vi "Util.Cmprs.LZW.CU_CompressUncompress__ogtk.vi"(8 "error in (no error)":errorcluster, 9 "LZWBits":i32, 10 "Data":u8[](array[numeric]) format="%.0x", 11 "Compress/Decompress (T/F)":bool) -> (0 "error out":errorcluster, 2 "Data out":u8[](array[numeric]) format="%.0x")   [LabVIEW 2020]
panel:
  # "LZW.CU_CompressUncompress.vi\n\nCompresses or Uncompresses data-stream according to the \"Lempel-Ziv-Welch\" compression algorithm\n\nPlease visit http://www.OpenG.org to learn about the\nOpen Source LabVIEW software movement.\n\nNOTICE -- YOU MUST LEAVE THIS NOTICE IN PLACE.  PER THE TERMS OF THE LICENSE BELOW, YOU MAY SUBLICENSE THIS SOFTWARE \nIN ANY WAY THAT DOES NOT CONFLICT WITH THIS LICENSE.\n\n### BSD License (http://www.opensource.org/licenses/bsd-license.php) Begin ###\n \nCopyright (c) 2007, Bill Clench <bclench@yahoo.com>\n\nAll rights reserved.\n\nRedistribution and use in source and binary forms, with or without modification, are permitted provided that the following conditions are met:\n\n    * Redistributions of source code must retain the above copyright notice, this list of conditions and the following disclaimer.\n    * Redistributions in binary form must reproduce the above copyright notice, this list of conditions and the following disclaimer in the \n       documentation and/or other materials provided with the distribution.\n    * Neither the name of SciWare, James Kring, Inc., nor the names of its contributors may be used to endorse or promote products derived \n       from this software without specific prior written permission.\n\nTHIS SOFTWARE IS PROVIDED BY THE COPYRIGHT HOLDERS AND CONTRIBUTORS \"AS IS\" AND ANY EXPRESS OR IMPLIED WARRANTIES, \nINCLUDING, BUT NOT LIMITED TO, THE IMPLIED WARRANTIES OF MERCHANTABILITY AND FITNESS FOR A PARTICULAR PURPOSE ARE \nDISCLAIMED. IN NO EVENT SHALL THE COPYRIGHT OWNER OR CONTRIBUTORS BE LIABLE FOR ANY DIRECT, INDIRECT, INCIDENTAL,\n SPECIAL, EXEMPLARY, OR CONSEQUENTIAL DAMAGES (INCLUDING, BUT NOT LIMITED TO, PROCUREMENT OF SUBSTITUTE GOODS OR \nSERVICES; LOSS OF USE, DATA, OR PROFITS; OR BUSINESS INTERRUPTION) HOWEVER CAUSED AND ON ANY THEORY OF LIABILITY, \nWHETHER IN CONTRACT, STRICT LIABILITY, OR TORT (INCLUDING NEGLIGENCE OR OTHERWISE) ARISING IN ANY WAY OUT OF THE USE \nOF THIS SOFTWARE, EVEN IF ADVISED OF THE POSSIBILITY OF SUCH DAMAGE.\n\n### BSD License End ###"
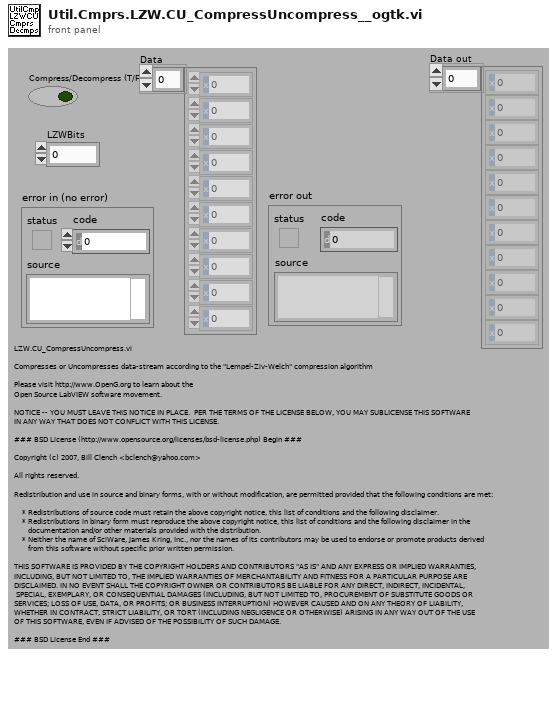
[diagram p1: front panel]
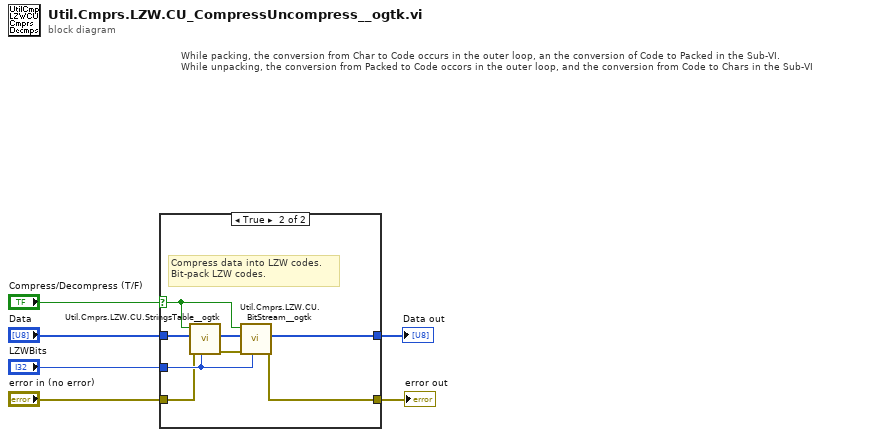
[diagram p0: block diagram]
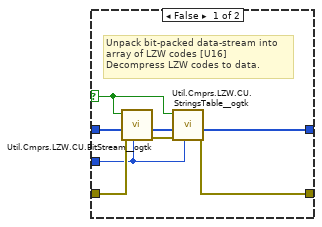
[diagram p2: hidden frame]
diagram:
  # "While packing, the conversion from Char to Code occurs in the outer loop, an the conversion of Code to Packed in the Sub-VI.\nWhile unpacking, the conversion from Packed to Code occors in the outer loop, and the conversion from Code to Chars in the Sub-VI"
  n1 = case shown="True" "Compress/Decompress (T/F)" {
    selector: "Compress/Decompress (T/F)" -> [w13 w22]
    tunnel: "Data" -> [w14 w19]
    tunnel: [w11 w21] -> w4
    tunnel: "LZWBits" -> [w9 w17]
    tunnel: "error in (no error)" -> [w10 w16]
    tunnel: [w7 w18] -> w1
    frame False {
      # "Unpack bit-packed data-stream into array of LZW codes [U16]\nDecompress LZW codes to data."
      n2 = call <userlib>:"Util.Cmprs.LZW.CU.BitStream__ogtk.vi"("Bits"=w9, "error in (no error)"=w10, "Chars in"=w14, "PackUnpack"=w13) -> ("error out"=w8:errorcluster, "Codes out"=w12:i16[])  [unwired: 5 in, 1 out]
      n3 = call <userlib>:"Util.Cmprs.LZW.CU.StringsTable__ogtk.vi"("Bits"=w9, "error in (no error)"=w8, "Codes in"=w12, "Pack"=w13) -> ("error out"=w7:errorcluster, "Chars out"=w11:u8[])  [unwired: 5 in, 1 out]
    }
    frame True {
      # "Compress data into LZW codes.\nBit-pack LZW codes."
      n4 = call <userlib>:"Util.Cmprs.LZW.CU.StringsTable__ogtk.vi"("Bits"=w17, "error in (no error)"=w16, "Chars in"=w19, "Pack"=w22) -> ("error out"=w15:errorcluster, "Codes out"=w20:i16[])  [unwired: 5 in, 1 out]
      n5 = call <userlib>:"Util.Cmprs.LZW.CU.BitStream__ogtk.vi"("Bits"=w17, "error in (no error)"=w15, "Codes in"=w20, "PackUnpack"=w22) -> ("error out"=w18:errorcluster, "Chars out"=w21:u8[])  [unwired: 5 in, 1 out]
    }
  }
  "Data out" <- w4
  "error out" <- w1
